vi "case-structure-calculator.vi"() -> ()   [LabVIEW 2025]
panel:
  out "result":dbl
  in  "a 2":dbl
  in  "a":dbl
  in  "Enum":enum16{"add", "multiply", "sub", "div"}(ring)
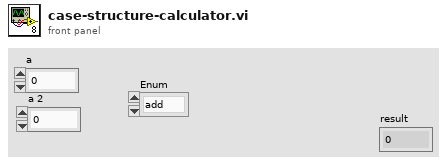
[diagram p1: front panel]
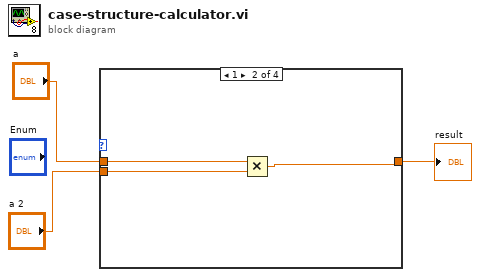
[diagram p0: block diagram]
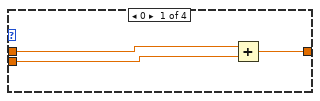
[diagram p2: hidden frame]
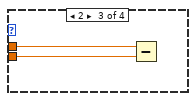
[diagram p3: hidden frame]
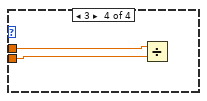
[diagram p4: hidden frame]
diagram:
  n1 = case shown="1" {
    selector: _ -> [_ _ _ _]
    tunnel: "a" -> [w6 w9 w12 w15]
    tunnel: "a 2" -> [w5 w8 w11 w14]
    tunnel: [w4 w7 _ _] -> w1
    frame 0 {
      n2 = Add(x=w6, y=w5) -> (x+y=w4:dbl)
    }
    frame 1 {
      n3 = Multiply(x=w9, y=w8) -> (x*y=w7:dbl)
    }
    frame 2 {
      n4 = Subtract(x=w12, y=w11) -> (x-y=w10:dbl)
    }
    frame 3 {
      n5 = Divide(x=w15, y=w14) -> (x/y=w13:dbl)
    }
  }
  "result" <- w1
